vi "GetUTCTimestamp.vi"() -> (3 "Timestamp":u64)   [LabVIEW 2018]
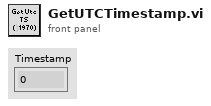
[diagram p1: front panel]
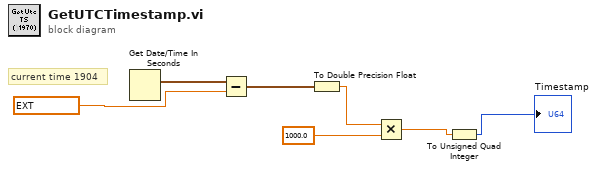
[diagram p0: block diagram]
diagram:
  # "current time 1904"
  n1 = Get Date/Time In Seconds() -> (seconds since 1Jan1904=w1:timestamp)
  n2 = Subtract(x=w1, y=ext 2082844800.0) -> (x-y=w2:timestamp)
  n3 = To Double Precision Float(number=w2) -> (double precision float=w3:dbl)
  n4 = Multiply(x=w3, y=1000.0) -> (x*y=w5:dbl)
  n5 = To Unsigned Quad Integer(1:w5) -> (0:→"Timestamp":u64)
